vi "Set pH&ISE Range.vi"(8 "error in (no error)":errorcluster, 9 "Range":enum16{"2000", "200"}(ring), 10 "Channel":T1, 11 "EPU452 in":refnum<class "EPU452.lvclass">) -> (0 "error out":errorcluster, 3 "EPU452 out":refnum<class "EPU452.lvclass">)   [LabVIEW 2018, in "EPU452.lvclass"]
uses:
  EPU452.lvclass
  Controls/Channels.ctl
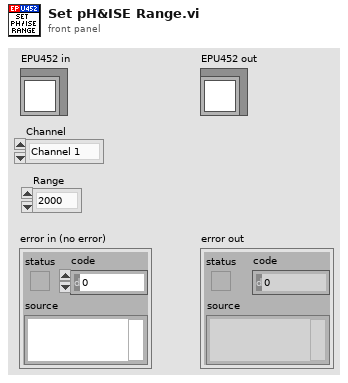
[diagram p1: front panel]
types:
  T1 = typedef "EPU452.lvclass/Channels.ctl" = enum16{"Channel 1", "Channel 2", "Channel 3", "Channel 4"}
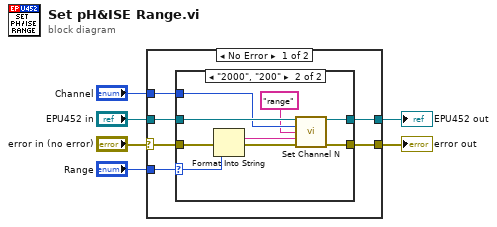
[diagram p0: block diagram]
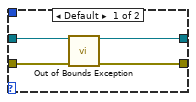
[diagram p2: hidden frame]
diagram:
  n1 = case shown="No Error" "error in (no error)" {
    selector: "error in (no error)" -> [w10 w27]
    tunnel: [w7 w27] -> w5
    tunnel: [w8 w26] -> w3
    tunnel: "EPU452 in" -> [w12 w26]
    tunnel: "Channel" -> [w11 _]
    tunnel: "Range" -> [w9 _]
    frame No Error {
      n2 = case shown="\"2000\", \"200\"" w9 {
        selector: w9 -> [_ w20]
        tunnel: w12 -> [w15 w25]
        tunnel: w11 -> [_ w24]
        tunnel: w10 -> [w16 w19]
        tunnel: [w14 w22] -> w8
        tunnel: [w13 w21] -> w7
        frame Default {
          n3 = call "Out of Bounds Exception.vi"("error in (no error)"=w16, "EPU452 in"=w15) -> ("error out"=w13:errorcluster, "EPU452 out"=w14:refnum<class "EPU452.lvclass">)  [unwired: 8 in]
        }
        frame "2000", "200" {
          n4 = Format Into String(error in=w19, w20) -> (resulting string=w17:string, error out=w18:errorcluster)  [unwired: 2 in]
          n5 = call "Set Channel N.vi"("EPU452 in"=w25, "Channel"=w24, "Function"="range", "Argument/s"=w17, "error in (no error)"=w18) -> ("EPU452 out"=w22:refnum<class "EPU452.lvclass">, "error out"=w21:errorcluster)  [unwired: 8 in, 1 out]
        }
      }
    }
    frame Error {
    }
  }
  "error out" <- w5
  "EPU452 out" <- w3
